vi "Find Local Msg Set.vi"(11 "TEMPLATE Actor in":refnum<class "TEMPLATE Actor.lvclass">) -> (3 "TEMPLATE Actor out":refnum<class "TEMPLATE Actor.lvclass">)   [LabVIEW 2025, in "_Template.lvlib" / "Templates.lvlib" / "TEMPLATE Actor.lvlib" / "TEMPLATE Actor.lvclass"]
uses:
  TEMPLATE Actor.lvclass
  C:/git/jettl/src/jettl/jettl/Actor/Actor.lvclass
  jettl/jettl/Actor/Actor.lvclass
  TEMPLATE Actor.lvclass/TEMPLATE Actor.ctl
  jettl/jettl/jettl.lvlib
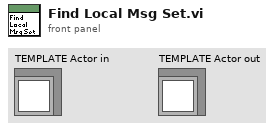
[diagram p1: front panel]
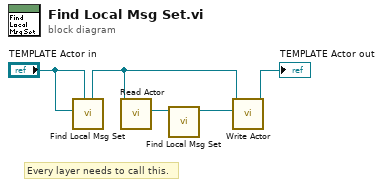
[diagram p0: block diagram]
diagram:
  # "Every layer needs to call this."
  n1 = call "Find Local Msg Set.vi"("Actor in"="TEMPLATE Actor in", "X Actor.lvclass"="TEMPLATE Actor in") -> ("Actor out"=w2:refnum<class "TEMPLATE Actor.lvclass">)  [unwired: 9 in]
  n2 = call-dynamic "Read Actor.vi"("TEMPLATE Actor in"=w2) -> ("Actor"=w5:refnum<class "Actor.lvclass">)  [unwired: 10 in]
  n3 = call-dynamic "Find Local Msg Set.vi"("Actor in"=w5) -> ("Actor out"=w4:refnum<class "Actor.lvclass">)  [unwired: 10 in]
  n4 = call-dynamic "Write Actor.vi"("Actor"=w4, "TEMPLATE Actor in"=w2) -> ("TEMPLATE Actor out"=→"TEMPLATE Actor out":refnum<class "TEMPLATE Actor.lvclass">)  [unwired: 9 in]
